vi "New BS120x Ethernet Device.vi"(5 "Auto-Refresh (T)":bool=TRUE, 6 "TCP port":u16=12345, 7 "Connect for Config Only? (F)":bool, 8 "error in (no error)":errorcluster, 9 "UDP port":u16=54321, 10 "Box IP address":string="192.168.1.100", 11 "Unit Type":T1) -> (0 "error out":errorcluster, 3 "BS120x Out":refnum<class "BS120x.lvclass">)   [LabVIEW 2021, in "BS120x Driver.lvlib"]
uses:
  BS120x Driver.lvlib
  ENET_BS1201/ENET_BS1201.lvclass
  ENET_BS1200/ENET_BS1200.lvclass
  ENET_BS120x/ENET_BS120x.lvclass
  C:/Users/Public/Documents/Projects/7100-00109 SW BS1201 LV Driver/trunk/source/ENET_BS120x/ENET_BS120x.lvclass
  C:/Users/Public/Documents/Projects/7100-00109 SW BS1201 LV Driver/trunk/source/BS120x.lvclass
  TypeDefs/UnitType.ctl
  BS120x.lvclass
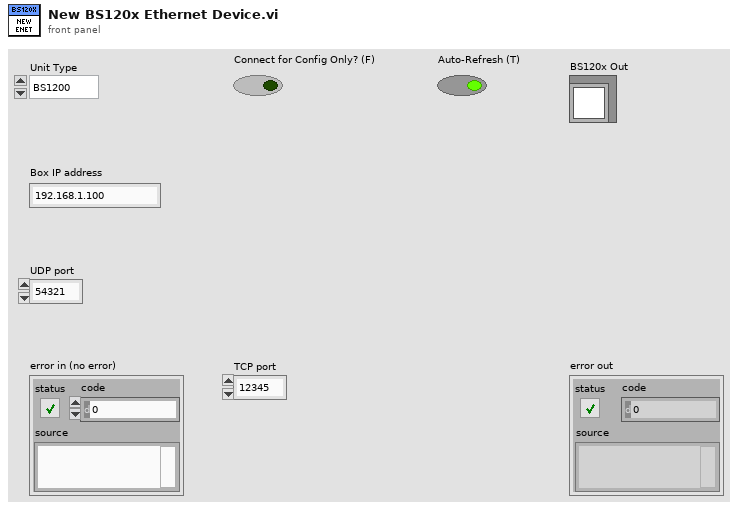
[diagram p1: front panel]
types:
  T1 = typedef "BS120x Driver.lvlib/BS120x.lvclass/UnitType.ctl" = enum16{"BS1200", "BS1201"}
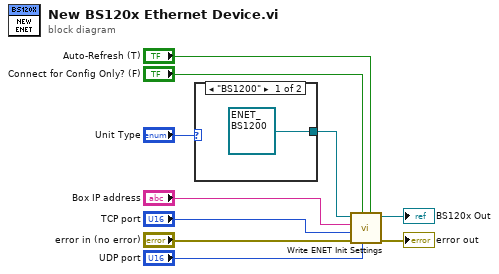
[diagram p0: block diagram]
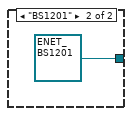
[diagram p2: hidden frame]
diagram:
  n1 = case shown="\"BS1200\"" "Unit Type" {
    tunnel: [refnum<class "ENET_BS1200.lvclass"> refnum ("BS120x Driver.lvlib:ENET_BS1200.lvclass") refnum<class "ENET_BS1201.lvclass"> refnum ("BS120x Driver.lvlib:ENET_BS1201.lvclass")] -> w9
    frame "BS1200" {
    }
    frame "BS1201" {
    }
  }
  n2 = call-dynamic "Write ENET Init Settings.vi"("Auto-Refresh (T)"="Auto-Refresh (T)", "UDP port"="UDP port", "Connect for Config Only? (F)"="Connect for Config Only? (F)", "error in (no error)"="error in (no error)", "TCP port"="TCP port", "Box IP address"="Box IP address", "Ethernet_BS1201 in"=w9) -> ("error out"=→"error out":errorcluster, "Ethernet_BS1201 out"=→"BS120x Out":refnum<class "ENET_BS120x.lvclass">)  [unwired: 3 in]
